vi "macro_PhotonVision_GetLatestTargets.vi"() -> ()   [LabVIEW 2019]
uses:
  PhotonVisionLib/SubVI/PhotonPipelineResult_Unpack.vi
  PhotonVisionLib/SubVI/PhotonPipelineResult_GetTargetCount.vi
  PhotonVisionLib/SubVI/PhotonPipelineResult_GetMetadata.vi
  PhotonVisionLib/SubVI/PhotonPipelineMetadata_GetAll.vi
  PhotonVisionLib/SubVI/Packet_decode_ByteI8.vi
  PhotonVisionLib/SubVI/PhotonTrackedTarget_Unpack.vi
  PhotonVisionLib/SubVI/PhotonMultiTargetPNPResult_unpack.vi
  PhotonVisionLib/SubVI/PhotonPipelineMetadata_Unpack.vi
  PhotonVisionLib/SubVI/PhotonPipelineResult_New.vi
  PhotonVisionLib/SubVI/Packet_decode_Flt64.vi
  PhotonVisionLib/SubVI/TargetCorner_New.vi
  PhotonVisionLib/SubVI/Packet_decode_Int32.vi
  PhotonVisionLib/SubVI/Packet_decode_Transform3d.vi
  PhotonVisionLib/SubVI/Packet_decode_Flt32.vi
  PhotonVisionLib/SubVI/Packet_decode_TargetCornerArray.vi
  PhotonVisionLib/SubVI/Packet_decode_Boolean.vi
  PhotonVisionLib/SubVI/PhotonPNPResult_unpack.vi
  PhotonVisionLib/SubVI/PhotonMultiTargetPNPResult_New.vi
  PhotonVisionLib/SubVI/Packet_decode_Int16.vi
  PhotonVisionLib/SubVI/Packet_decode_Int64.vi
  <vilib>/Rock Robotics/WPI/ThirdParty/JAS_Junk/TrajLib/VI/Transform3d_Create_Trans3dRot3d.vi
  <vilib>/Rock Robotics/WPI/ThirdParty/JAS_Junk/TrajLib/VI/Translation3d_Create.vi
  <vilib>/Rock Robotics/WPI/ThirdParty/JAS_Junk/TrajLib/VI/Rotation3d_Create_Quaternion.vi
  <vilib>/Rock Robotics/WPI/ThirdParty/JAS_Junk/TrajLib/VI/Quaternion_New.vi
  PhotonVisionLib/SubVI/PhotonPNPResult_New.vi
  <vilib>/Rock Robotics/WPI/ThirdParty/JAS_Junk/TrajLib/VI/Quaternion_Normalize.vi
  <vilib>/Rock Robotics/WPI/ThirdParty/JAS_Junk/TrajLib/VI/Quaternion_New_Default.vi
  <vilib>/Rock Robotics/Network Tables/NT Read Value.vi
  <vilib>/Rock Robotics/Network Tables/NT Read Raw.vi
  PhotonVisionLib/PhotonVisionLib.lvlib
  <vilib>/Rock Robotics/WPI/ThirdParty/JAS_Junk/TrajLib/Trajectory_Library.lvlib
panel:
  out "TargetFound":bool
  out "Yaw Offset (Degrees)":dbl
  out "DistanceToTarget (Meters)":dbl
  in  "Gyro Reading (Deg)":dbl
  in  "Drive Encoder  Dstance (Meters)":dbl
  out "IsConnected":bool
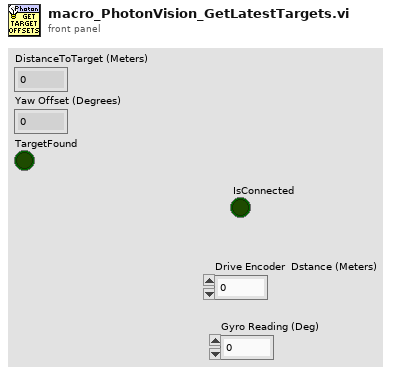
[diagram p1: front panel]
types:
  T1 = typedef "PhotonVisionLib.lvlib/PhotonPipelineResultType.ctl" = cluster{"Targets":T2[], "PhotonMultiTargetPNPResult":T8, "PhotonPipelineMetadata":T10}
  T2 = typedef "PhotonVisionLib.lvlib/PhotonTrackedTargetType.ctl" = cluster{"Yaw":dbl, "Pitch":dbl, "Area":dbl, "Skew":dbl, "MinAreaRectCorners":T3[], "BestCameraToTarget":T4, "FiducialId":i32, "AltCameraToTarget":T4, "PoseAmbiguity":dbl, "DetectedCorners":T3[], "ObjDetectId":i32, "ObjDetectConf":sgl}
  T3 = typedef "PhotonVisionLib.lvlib/TargetCornerType.ctl" = cluster{"X":dbl, "Y":dbl}
  T4 = typedef "Trajectory_Library.lvlib/TRANSFORM3D.ctl" = cluster{"TRANSLATION3D":T5, "ROTATION3D":T6, "XF":bool}
  T5 = typedef "Trajectory_Library.lvlib/TRANSLATION3D.ctl" = cluster{"X":dbl, "Y":dbl, "Z":dbl}
  T6 = typedef "Trajectory_Library.lvlib/ROTATION3D.ctl" = cluster{"Q_quaternion":T7}
  T7 = typedef "Trajectory_Library.lvlib/QUATERNION.ctl" = cluster{"R":dbl, "V":dbl[]}
  T8 = typedef "PhotonVisionLib.lvlib/PhotonMultiTargetPNPResultType.ctl" = cluster{"PhotonPNPResult":T9, "FiducialIDsUsed":i16[]}
  T9 = typedef "PhotonVisionLib.lvlib/PhotonPNPResultType.ctl" = cluster{"IsPresent":bool, "bestReprojErr":dbl, "altReprojErr":dbl, "ambiguity":dbl, "Best":T4, "Alt":T4}
  T10 = typedef "PhotonVisionLib.lvlib/PhotonPipelineMetadataType.ctl" = cluster{"CaptureTimestampMicros":i64, "PublishTimestampMicros":i64, "SequenceID":i64, "TimeSinceLastPong":i64}
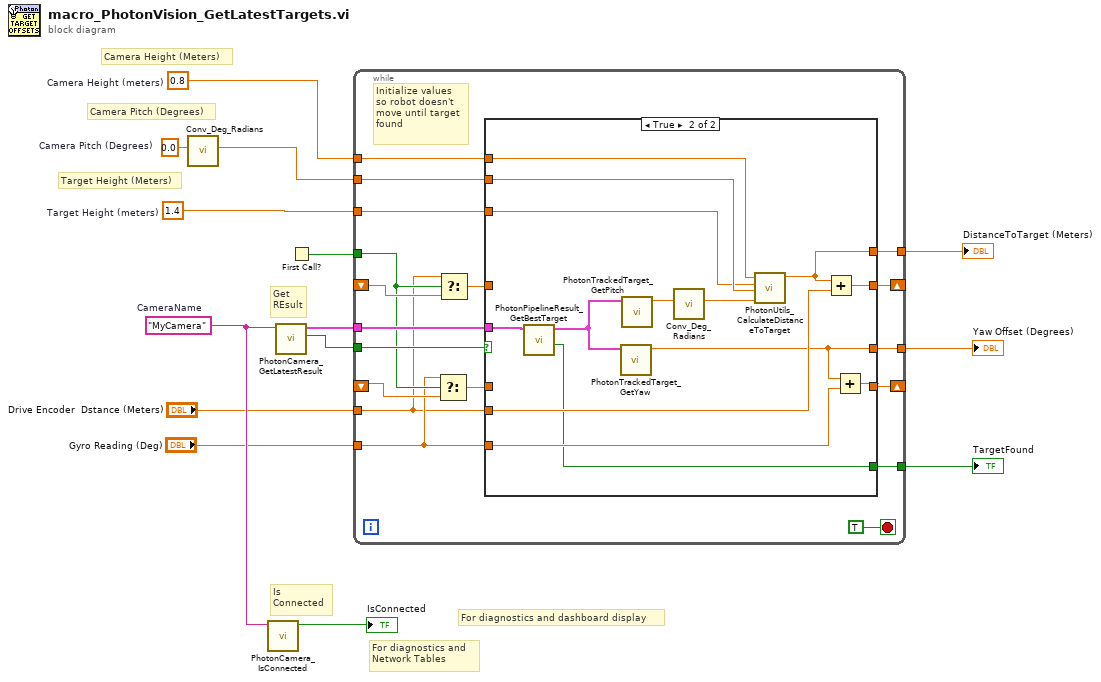
[diagram p0: block diagram]
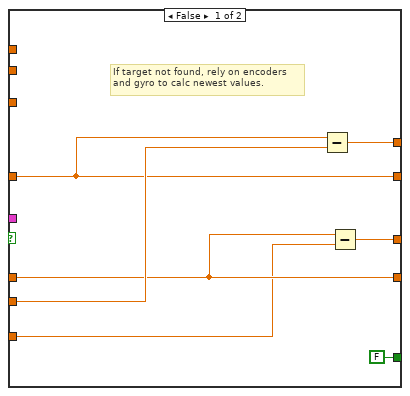
[diagram p2: hidden frame]
diagram:
  w7 = 1.4  # Target Height (meters)
  w9 = 0.8  # Camera Height (meters)
  w12 = 0.0  # Camera Pitch (Degrees)
  w14 = "MyCamera"  # CameraName
  # "For diagnostics and dashboard display"
  # "Camera Pitch (Degrees)"
  # "Target Height (Meters)"
  # "Camera Height (Meters)"
  # "For diagnostics and \nNetwork Tables"
  # "Is\nConnected"
  # "Get\nREsult"
  n1 = call <vilib>:"Conv_Deg_Radians.vi"("Degress"=w12) -> ("Radians"=w8:dbl)  [unwired: 10 in]
  n2 = call "PhotonCamera_IsConnected.vi"("CameraName"=w14) -> ("IsConnected"=→"IsConnected":bool)  [unwired: 9 in, 1 out]
  n3 = call "PhotonCamera_GetLatestResult.vi"("CameraName"=w14) -> ("HasTargets"=w11:bool, "PipelineResult"=w10:T1)  [unwired: 6 in, 3 out]
  n4 = First Call?() -> (First Call?: T/F=w2:bool)
  n5 = while {
    tunnel: w11 -> [w32]
    tunnel: w10 -> [w31]
    tunnel: w9 -> [w30]
    tunnel: w8 -> [w29]
    tunnel: w7 -> [w28]
    tunnel: [w27] -> w6
    tunnel: [w26] -> w5
    tunnel: "Drive Encoder  Dstance (Meters)" -> [w15]
    shift-right: [w24] -> _
    shift-left: _ -> [w22]
    tunnel: "Gyro Reading (Deg)" -> [w16]
    shift-right: [w23] -> _
    shift-left: _ -> [w20]
    tunnel: w2 -> [w18]
    tunnel: [w17] -> w1
    stop <- TRUE stop-if-true
    # "Initialize values\nso robot doesn't\nmove until target\nfound"
    n6 = Select(t=w16, s=w18, f=w20) -> (s? t:f=w19:dbl)
    n7 = Select(t=w15, s=w18, f=w22) -> (s? t:f=w21:dbl)
    n8 = case shown="True" w32 {
      tunnel: w31 -> [_ w53]
      tunnel: [w36 w43] -> w26
      tunnel: w30 -> [_ w49]
      tunnel: w29 -> [_ w48]
      tunnel: w28 -> [_ w47]
      tunnel: [w38 w46] -> w27
      tunnel: w15 -> [w39 w45]
      tunnel: [w37 w44] -> w24
      tunnel: w21 -> [w37 _]
      tunnel: w16 -> [w34 w42]
      tunnel: [w35 w41] -> w23
      tunnel: w19 -> [w35 _]
      tunnel: [FALSE ("TargetFound") w40] -> w17
      frame False {
        # "If target not found, rely on encoders\nand gyro to calc newest values."
        n9 = Subtract(x=w37, y=w39) -> (x-y=w38:dbl)
        n10 = Subtract(x=w35, y=w34) -> (x-y=w36:dbl)
      }
      frame True {
        n11 = call "PhotonPipelineResult_GetBestTarget.vi"("PhotonPipelineResult"=w53) -> ("TargetFound"=w40:bool, "PhotonTrackedTarget"=w52:T2)  [unwired: 9 in]
        n12 = call "PhotonTrackedTarget_GetYaw.vi"("TrackedTarget"=w52) -> ("Yaw"=w43:dbl)  [unwired: 10 in]
        n13 = call "PhotonTrackedTarget_GetPitch.vi"("TrackedTarget"=w52) -> ("Pitch"=w51:dbl)  [unwired: 10 in]
        n14 = call <vilib>:"Conv_Deg_Radians.vi"("Degress"=w51) -> ("Radians"=w50:dbl)  [unwired: 10 in]
        n15 = call "PhotonUtils_CalculateDistanceToTarget.vi"("TargetPitch_Radians"=w50, "CameraPitch_Radians"=w48, "TargetHeight_Meters"=w47, "CameraHeight_Meters"=w49) -> ("DistanceToTarget_Meters"=w46:dbl)  [unwired: 7 in]
        n16 = Add(x=w46, y=w45) -> (x+y=w44:dbl)
        n17 = Add(x=w43, y=w42) -> (x+y=w41:dbl)
      }
    }
  }
  "DistanceToTarget (Meters)" <- w6
  "Yaw Offset (Degrees)" <- w5
  "TargetFound" <- w1
